vi "editscenario format Post to Conditions.vi"(11 "Save POST":T3) -> (3 "Conditions":T1[](array[typedef]))   [LabVIEW 2011]
uses:
  ITK EXT/utils/keyedarr.llb/Keyed Array.ctl
  server/database/Scenarios/Conditions/Condition Record.ctl
  server/database/Scenarios/Conditions/Condition Operators.ctl
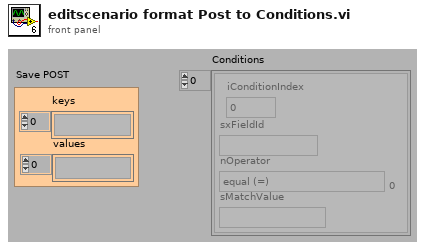
[diagram p1: front panel]
types:
  T1 = typedef "Condition Record.ctl" = cluster{"iConditionIndex":i32, "sxFieldId":string, "nOperator":T2, "sMatchValue":string}
  T2 = typedef "Condition Operators.ctl" = enum16{"equal (=)", "not equal (\\u2260)", "less than (<)", "less than or equal (\\u2264)", "greater than (>)", "greater than or equal (\\u2265)", "contains", "does not contain"}
  T3 = typedef "Keyed Array.ctl" = cluster{"keys":string[], "values":string[]}
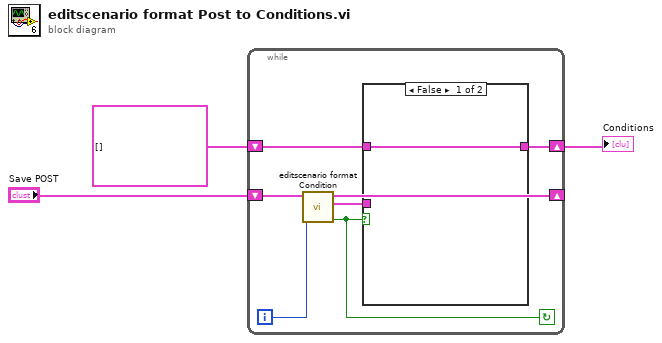
[diagram p0: block diagram]
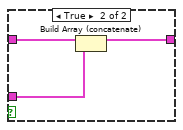
[diagram p2: hidden frame]
diagram:
  n1 = while {
    shift-right: [w8] -> _
    shift-left: "Save POST" -> [w10]
    shift-right: [w4] -> w2
    shift-left: T1[] [] -> [w7]
    i -> [w9]
    stop <- w6 continue-if-true
    n2 = call "editscenario format Condition.vi"("Index (0)"=w9, "POST (empty)"=w10) -> ("Valid Condition?"=w6:bool, "Condition"=w5:T1, "POST out"=w8:T3)  [unwired: 7 out]
    n3 = case shown="False" w6 {
      tunnel: w7 -> [w11 w13]
      tunnel: w5 -> [_ w14]
      tunnel: [w11 w12] -> w4
      frame False {
      }
      frame True {
        n4 = Build Array (concatenate)(w13, w14) -> (w12:T1[])
      }
    }
  }
  "Conditions" <- w2
